vi "Download zip file.vi"(0 "client handle":T1, 5 "Standalone?":bool, 7 "Artifactory ZIP Directory":string, 9 "Save Path":path=path "C:/Automation/APLs", 11 "Error In":errorcluster) -> (4 "client handle out":T1, 6 "Output Path":path, 15 "Error Out":errorcluster)   [LabVIEW 2016]
uses:
  <vilib>/httpClient/ClientHandle.ctl
  <vilib>/regexp/Match Regular Expression.xnode
  <vilib>/httpClient/LabVIEWHTTPClient.lvlib
  <vilib>/zip/NI_Unzip.lvlib
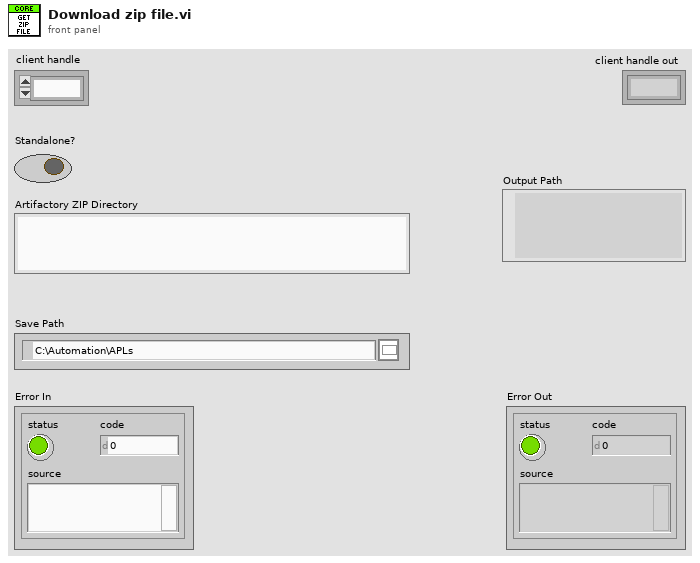
[diagram p1: front panel]
types:
  T1 = typedef "LabVIEWHTTPClient.lvlib/ClientHandle.ctl" = refnum<k1>
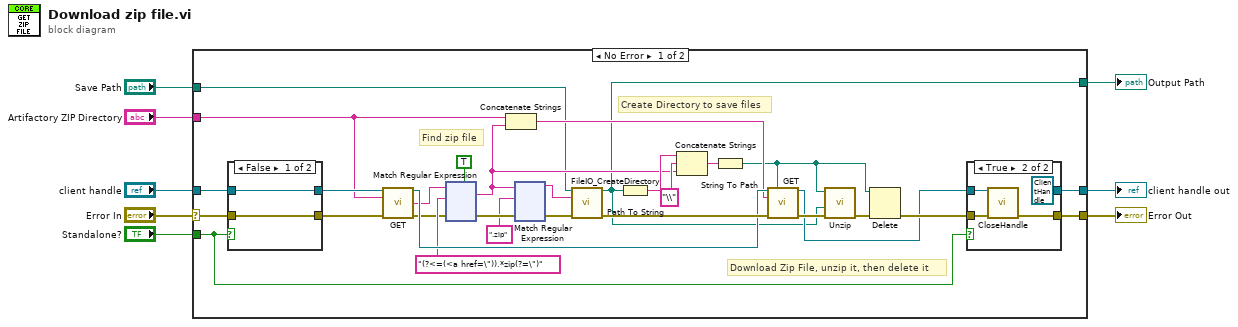
[diagram p0: block diagram]
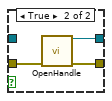
[diagram p3: hidden frame]
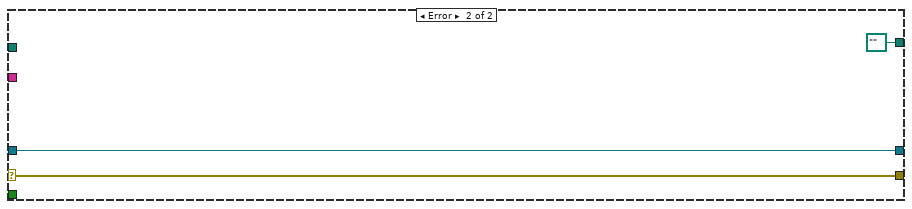
[diagram p4: hidden frame]
diagram:
  n1 = case shown="No Error" "Error In" {
    selector: "Error In" -> [w34 w280]
    tunnel: "client handle" -> [w38 w279]
    tunnel: [w37 w279] -> w7
    tunnel: "Standalone?" -> [w36 _]
    tunnel: [w35 w280] -> w5
    tunnel: "Artifactory ZIP Directory" -> [w15 _]
    tunnel: [w10 path ""] -> w2
    tunnel: "Save Path" -> [w11 _]
    frame No Error {
      # "Create Directory to save files"
      # "Find zip file"
      # "Download Zip File, unzip it, then delete it"
      n2 = case shown="False" w36 {
        tunnel: [w274 w277] -> w16
        tunnel: w38 -> [w274 _]
        tunnel: w34 -> [w273 w276]
        tunnel: [w273 w275] -> w17
        frame False {
        }
        frame True {
          n3 = call <vilib>:"OpenHandle.vi"("error in (no error)"=w276) -> ("client handle out"=w277:T1, "error out"=w275:errorcluster)  [unwired: 13 in]
        }
      }
      n4 = call <vilib>:"GET.vi"("client handle"=w16, "url"=w15, "error in (no error)"=w17) -> ("client handle out"=w23:T1, "body"=w20:string, "error out"=w19:errorcluster)  [unwired: 9 in, 1 out]
      n5 = xnode "Match Regular Expression"("input string"=w20, "regular expression"="(?<=(<a href=\")).*zip(?=\")", "error in"=w19, "multiline? (F)"=TRUE) -> ("whole match"=w29:string, "error out"=w26:errorcluster)  [unwired: 2 in, 3 out]
      n6 = Concatenate Strings(w15, w29) -> (w22:string)
      n7 = xnode "Match Regular Expression"("input string"=w29, "regular expression"=".zip", "error in"=w26) -> ("before match"=w28:string, "error out"=w27:errorcluster)  [unwired: 3 in, 3 out]
      n8 = call "FileIO_CreateDirectory.vi"("Base Path"=w11, "Directory Name"=w28, "Error In"=w27) -> ("File Path Control"=w10:path, "Error Out"=w24:errorcluster)  [unwired: 11 in]
      n9 = Path To String(path=w10) -> (string=w33:string)
      n10 = Concatenate Strings(w33, "\\" ("string"), w29) -> (w31:string)
      n11 = String To Path(string=w31) -> (path=w9:path)
      n12 = call <vilib>:"GET.vi"("client handle"=w23, "output file"=w9, "url"=w22, "error in (no error)"=w24) -> ("client handle out"=w12:T1, "error out"=w13:errorcluster)  [unwired: 8 in, 2 out]
      n13 = call <vilib>:"Unzip.vi"("error in (no error)"=w13, "Target directory (same as Zip file if empty)"=w10, "Zip file"=w9) -> ("error out"=w32:errorcluster)  [unwired: 6 in, 2 out]
      n14 = Delete(path (use dialog)=w9, error in=w32) -> (error out=w14:errorcluster)  [unwired: 3 in, 2 out]
      n15 = case shown="True" w36 {
        tunnel: [w268 T1 refnum ("client handle out")] -> w37
        tunnel: w12 -> [w268 w270]
        tunnel: w14 -> [w267 w272]
        tunnel: [w267 w271] -> w35
        frame False {
        }
        frame True {
          n16 = call <vilib>:"CloseHandle.vi"("client handle"=w270, "error in (no error)"=w272) -> ("error out"=w271:errorcluster)  [unwired: 13 in]
        }
      }
    }
    frame Error {
    }
  }
  "Error Out" <- w5
  "Output Path" <- w2
  "client handle out" <- w7
